vi "Tosca-End On Rep Boundary.vi"(0 "Queue in":refnum<queue>, 7 "Stim data in":T1) -> (4 "Queue out":refnum<queue>, 15 "error out":errorcluster)   [LabVIEW 2020]
uses:
  Typedefs/Tosca-State AODO.ctl
  epl-vi-lib/Signal Synthesis VIs/4th Generation/Classes/SignalManager/SignalManager.lvclass
  Typedefs/Tosca-AO Runtime.ctl
  Typedefs/Tosca-DO Runtime.ctl
  Typedefs/Tosca-AODO Data.ctl
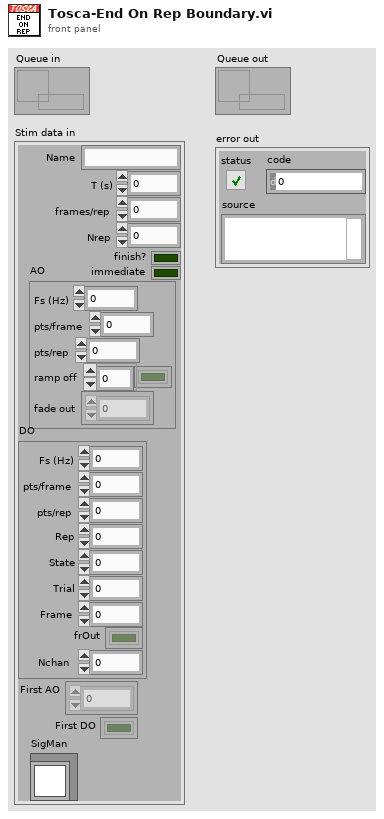
[diagram p1: front panel]
types:
  T1 = typedef "Tosca-State AODO.ctl" = cluster{"Name":string, "T (s)":dbl, "First AO":dbl[][], "frames/rep":i32, "finish?":bool, "Nrep":i32, "AO":T2, "DO":T3, "immediate":bool, "First DO":bool[][], "SigMan":refnum<class "SignalManager.lvclass">}
  T2 = typedef "Tosca-AO Runtime.ctl" = cluster{"Fs (Hz)":dbl, "pts/frame":i32, "pts/rep":i32, "ramp off":bool[], "fade out":dbl[][]}
  T3 = typedef "Tosca-DO Runtime.ctl" = cluster{"Fs (Hz)":dbl, "pts/frame":i32, "pts/rep":i32, "Rep":i32, "State":i32, "Trial":i32, "Frame":i32, "frOut":bool[], "Nchan":i32}
  T4 = typedef "Tosca-AODO Data.ctl" = cluster{"AO":dbl[][], "DO":bool[][], "frame":i32, "stop":bool}
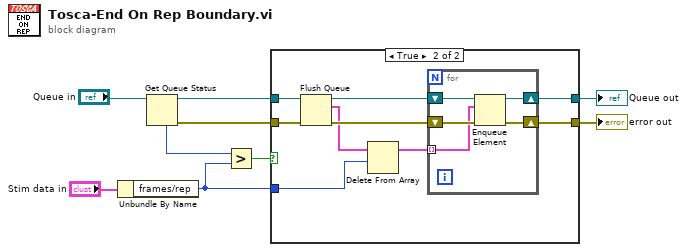
[diagram p0: block diagram]
diagram:
  n1 = Unbundle By Name("Stim data in") -> ("frames/rep"=w1:i32)
  n2 = Get Queue Status(queue="Queue in") -> (queue out=w4:refnum<queue>, error out=w3:errorcluster, # elements in queue=w5:i32)  [unwired: 2 in, 5 out]
  n3 = Greater?(x=w5, y=w1) -> (0:w2:bool)
  n4 = case shown="True" w2 {
    tunnel: [w11 w18] -> w9
    tunnel: [w10 w17] -> w8
    tunnel: w4 -> [w11 w16]
    tunnel: w3 -> [w10 w15]
    tunnel: w1 -> [_ w13]
    frame False {
    }
    frame True {
      n5 = Flush Queue(queue=w16, error in (no error)=w15) -> (queue out=w20:refnum<queue>, remaining elements=w14:T4[], error out=w19:errorcluster)
      n6 = Delete From Array(array=w14, length=w13) -> (array with subset deleted=w12:T4[])  [unwired: 1 in, 1 out]
      n7 = for {
        shift-right: [w23] -> w18
        shift-left: w20 -> [w25]
        shift-right: [w22] -> w17
        shift-left: w19 -> [w24]
        tunnel: w12 -> [w21] mode=indexing
        n8 = Enqueue Element(queue=w25, element=w21, error in (no error)=w24) -> (queue out=w23:refnum<queue>, error out=w22:errorcluster)  [unwired: 1 in, 1 out]
      }
    }
  }
  "error out" <- w8
  "Queue out" <- w9
